vi "setDataSize.vi"(8 "error in (no error)":errorcluster, 10 "acquisition count":i32, 11 "CCD in":refnum<class "CCD.lvclass">) -> (0 "error out":errorcluster, 1 "ID":i32, 2 "results-JSON string":string, 3 "CCD out":refnum<class "CCD.lvclass">)   [LabVIEW 2023, in "CCD.lvclass"]
uses:
  CCD.lvclass
  CCD.lvclass/CCD.ctl
  20f7d3bd-08ac-4524-9bed-df36c1da25a0.vi
  GenericDevice/GenericDevice.lvclass
  cab240a6-cbf4-4e2c-ab79-96d9c1b88265.vi
  <vilib>/IlluminatedG/lv-web-crypto/lv-json/JSON/JSON.lvlib
panel:
  # "Connector Pane"
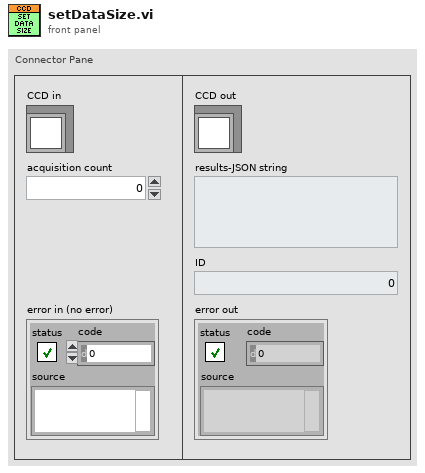
[diagram p1: front panel]
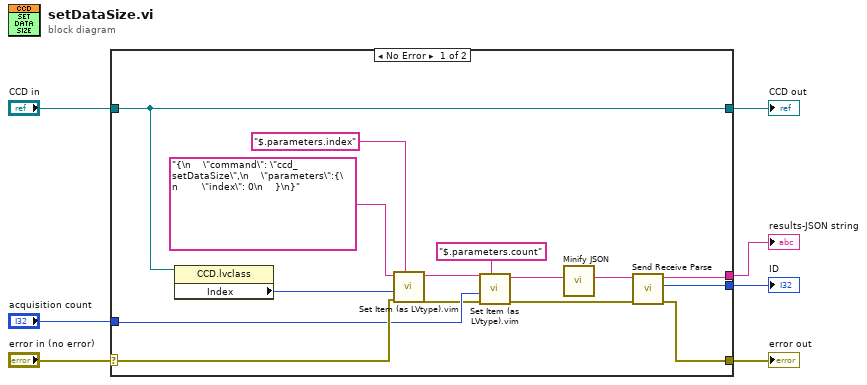
[diagram p0: block diagram]
diagram:
  n1 = case shown="No Error" "error in (no error)" {
    selector: "error in (no error)" -> [w18 w24]
    tunnel: [w12 w24] -> w6
    tunnel: [w20 w23] -> w4
    tunnel: "CCD in" -> [w20 w23]
    tunnel: "acquisition count" -> [w16 _]
    tunnel: [w11 _] -> w3
    tunnel: [w10 _] -> w2
    frame No Error {
      n2 = property class="CCD.lvclass"(reference=w20) -> ("Index"=w19:i32)  [unwired: 1 in, 2 out]
      n3 = call "Set Item (as LVtype).vim"("$Path or Item Name"="$.parameters.index", "error in (no error)"=w18, "Anything"=w19, "JSON"="{\n    \"command\": \"ccd_setDataSize\",\n    \"parameters\":{\n        \"index\": 0\n    }\n}") -> ("error out"=w15:errorcluster, "<JSON>"=w13:string)  [unwired: 4 in, 1 out]
      n4 = call "Set Item (as LVtype).vim"("$Path or Item Name"="$.parameters.count", "error in (no error)"=w15, "Anything"=w16, "JSON"=w13) -> ("error out"=w14:errorcluster, "<JSON>"=w9:string)  [unwired: 4 in, 1 out]
      n5 = call <vilib>:"Minify JSON.vi"("JSON String"=w9) -> ("Minified JSON"=w8:string)  [unwired: 10 in]
      n6 = call "Send Receive Parse.vi"("error in"=w14, "<JSON>"=w8) -> ("error out"=w12:errorcluster, "ID"=w10:i32, "results-JSON string"=w11:string)  [unwired: 7 in]
    }
    frame Error {
    }
  }
  "error out" <- w6
  "CCD out" <- w4
  "results-JSON string" <- w3
  "ID" <- w2
